vi "GetCameraImage.vi"(8 "error in (no error)":errorcluster, 10 "Get Image (-1: latest)":i32=-1, 11 "Microscope":refnum<class "Microscope.lvclass">) -> (0 "error out":errorcluster, 1 "Coords":T1, 2 "image data":T2, 3 "Microscope out":refnum<class "Microscope.lvclass">)   [LabVIEW 2013, in "Microscope.lvclass"]
doc: "---------------------------------------------------------------\nJKI State Machine Objects™\nhttp://jki.net/state-machine-objects/\nCopyright (C) 2005-2015, JKI <info@jki.net>\nALL RIGHTS RESERVEDJKI State Machine Objects (SMO) 1.0.0.4\nJKI - JKI\nCopyright (c) 2015, JKI"
uses:
  Microscope.lvclass
  Camera/Camera.lvclass
  <vilib>/picture/picture.llb/imagedata.ctl
  XYStage/Typedefs/(real)Coords--Cluster.ctl
  XYStage/XYStage.lvclass
panel:
  # "For instructions on how to use the JKI State Machine Objects, examples and video tutorials, visit:\nhttp://jki.net/state-machine-objects/\n\nJKI State Machine Objects™\nhttp://jki.net/state-machine-objects/\nCopyright (C) 2005-2015, JKI <info@jki.net>\nALL RIGHTS RESERVED"
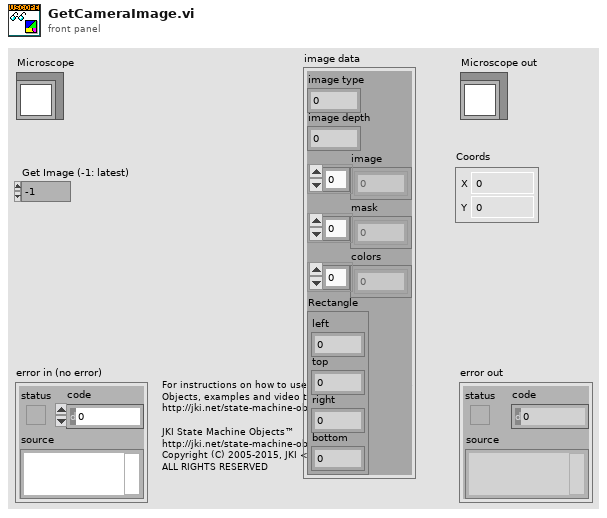
[diagram p1: front panel]
types:
  T1 = typedef "XYStage.lvclass/(real)Coords--Cluster.ctl" = cluster{"X":dbl, "Y":dbl}
  T2 = typedef "imagedata.ctl" = cluster{"image type":i32, "image depth":i32, "image":u8[], "mask":u8[], "colors":u32[], "Rectangle":cluster{"left":i16, "top":i16, "right":i16, "bottom":i16}}
  T3 = typedef "Microscope.lvclass/Dependencies--Cluster.ctl" = cluster{"XYStage":refnum<class "XYStage.lvclass">, "Camera":refnum<class "Camera.lvclass">}
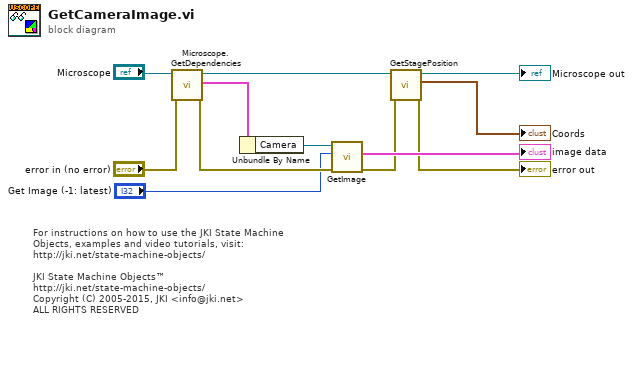
[diagram p0: block diagram]
diagram:
  # "For instructions on how to use the JKI State Machine Objects, examples and video tutorials, visit:\nhttp://jki.net/state-machine-objects/\n\nJKI State Machine Objects™\nhttp://jki.net/state-machine-objects/\nCopyright (C) 2005-2015, JKI <info@jki.net>\nALL RIGHTS RESERVED"
  n1 = call "Microscope.GetDependencies.vi"("error in (no error)"="error in (no error)", "Microscope"="Microscope") -> ("error out"=w8:errorcluster, "Dependencies"=w10:T3, "Microscope out"=w5:refnum<class "Microscope.lvclass">)  [unwired: 7 in]
  n2 = Unbundle By Name(w10) -> ("Camera"=w9:refnum<class "Camera.lvclass">)
  n3 = call "GetImage.vi"("error in (no error)"=w8, "Get Image (-1: latest)"="Get Image (-1: latest)", "Camera"=w9) -> ("error out"=w3:errorcluster, "image data"=→"image data":T2)  [unwired: 6 in, 1 out]
  n4 = call "GetStagePosition.vi"("error in (no error)"=w3, "Microscope"=w5) -> ("error out"=→"error out":errorcluster, "Coords"=→"Coords":T1, "Microscope out"=→"Microscope out":refnum<class "Microscope.lvclass">)  [unwired: 7 in]
